vi "IIR Filter Design.vi"() -> ()   [LabVIEW 2020]
doc: "Displays the Transfer Function of the filter selected from the front panel controls. \n\nYou can select any of the 5 IIR filter design methods (Bessel, Butterworth, Chebyshev I and II, and Elliptic) and the passband type (lowpass, highpass, bandpass, and bandstop)."
uses:
  <vilib>/Analysis/3filter.llb/Filter Passband Type.ctl
  <vilib>/Utility/error.llb/DialogType.ctl
  <vilib>/Analysis/NI_AALPro.lvlib
  <vilib>/measure/NI_MAPro.lvlib
  <vilib>/Analysis/NI_AALBase.lvlib
panel:
  out "Error Message":string
  in  "filter type":T1
  in  "Stop":bool
  in  "sampling rate":dbl=1000.0 format="%#.6g"
  in  "Attenuation":dbl(slide)=40.0 scale=0.0..150.0
  in  "Ripple":dbl(slide)=0.1 scale=0.0..1.0
  in  "high cutoff frequency":dbl(slide)=300.0 scale=0.0..500.0
  in  "low cutoff frequency":dbl(slide)=100.0 scale=0.0..500.0
  in  "Order":i32(slide)=4 scale=0.0..10.0
  in  "Filter Design":T2(ring)
  out "Phase Response":cluster{dbl, dbl, dbl[]}(graph)
  out "Magnitude Response":cluster{dbl, dbl, dbl[]}(graph)
  # "Overview: Demonstrates the design options for IIR filters.\nRequirements: LabVIEW Full Development System\nInstructions:\n1. Run the VI.\n2. Manipulate the parameters and observe the results in the Magnitude Response and Phase Response graphs.\n3. Click Stop to stop the VI."
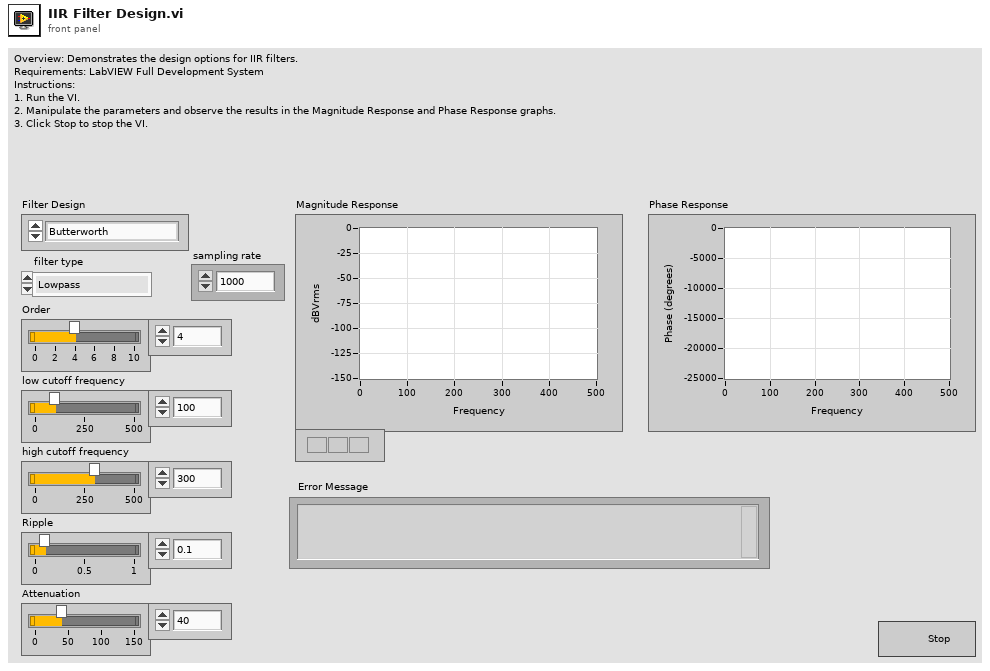
[diagram p1: front panel]
types:
  T1 = typedef "NI_AALBase.lvlib/Filter Passband Type.ctl" = enum32{"Lowpass", "Highpass", "Bandpass", "Bandstop"}
  T2 = enum16{"Butterworth", "Chebyshev", "Inverse Chebyshev", "Elliptic", "Bessel"}
  T3 = enum32{"Vrms", "Vpk", "Vrms^2", "Vpk^2", "Vrms/rtHz", "Vpk/rtHz", "Vrms^2/Hz", "Vpk^2/Hz"}
  T4 = enum16{"Power (Vrms^2)", "Amplitude (Vrms)", "Gain (amplitude ratio)"}
  T5 = typedef "DialogType.ctl" = u16
  T6 = cluster{"filter structure":enum32{"IIR 2nd Order", "IIR 4th Order"}, "Reverse Coefficients":dbl[], "Forward Coefficients":dbl[]}
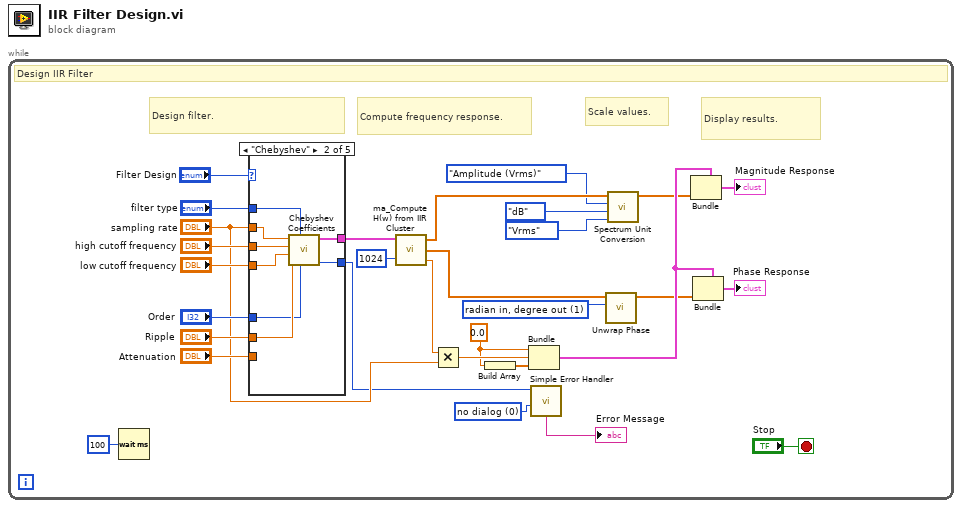
[diagram p0: block diagram]
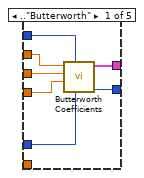
[diagram p2: hidden frame]
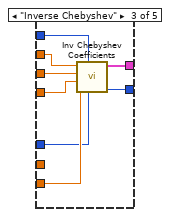
[diagram p3: hidden frame]
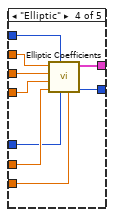
[diagram p4: hidden frame]
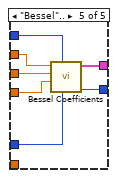
[diagram p5: hidden frame]
diagram:
  n1 = while {
    stop <- "Stop" stop-if-true
    w1 = 0.0
    w3 = T5 0 items=["no dialog", "OK message", "continue or stop message", "OK message + warnings", "continue/stop + warnings"] ("type of dialog (OK msg:1)")
    w10 = 1 items=["radian in, radian out", "radian in, degree out", "degree in, degree out", "degree in, radian out"] ("phase unit")
    # "Display results."
    # "Scale values."
    # "Compute frequency response."
    # "Design filter."
    # "Design IIR Filter"
    n2 = Wait (ms)(milliseconds to wait=u32 100) -> ()  [unwired: 1 out]
    n3 = case shown="\"Chebyshev\"" "Filter Design" {
      tunnel: "filter type" -> [w32 w45 w53 w60 w69]
      tunnel: "high cutoff frequency" -> [w37 w44 w52 w62 w68]
      tunnel: "low cutoff frequency" -> [w36 w43 w51 w61 w67]
      tunnel: "Order" -> [w35 w41 w49 w57 w66]
      tunnel: "Ripple" -> [_ w42 _ w59 _]
      tunnel: "Attenuation" -> [_ _ w50 w56 _]
      tunnel: "sampling rate" -> [w34 w40 w48 w58 w65]
      tunnel: [w33 w39 w47 w55 w64] -> w14
      tunnel: [w31 w38 w46 w54 w63] -> w2
      frame .."Butterworth" {
        n4 = call <vilib>:"Butterworth Coefficients.vi"("order"=w35, "filter type"=w32, "low cutoff freq: fl"=w36, "high cutoff freq: fh"=w37, "sampling freq: fs"=w34) -> ("error"=w31:i32, "IIR Filter Cluster"=w33:T6)  [unwired: 5 in]
      }
      frame "Chebyshev" {
        n5 = call <vilib>:"Chebyshev Coefficients.vi"("order"=w41, "filter type"=w45, "ripple(dB)"=w42, "low cutoff freq: fl"=w43, "high cutoff freq: fh"=w44, "sampling freq: fs"=w40) -> ("error"=w38:i32, "IIR Filter Cluster"=w39:T6)  [unwired: 4 in]
      }
      frame "Inverse Chebyshev" {
        n6 = call <vilib>:"Inv Chebyshev Coefficients.vi"("order"=w49, "filter type"=w53, "attenuation (dB)"=w50, "low cutoff freq: fl"=w51, "high cutoff freq: fh"=w52, "sampling freq: fs"=w48) -> ("error"=w46:i32, "IIR Filter Cluster"=w47:T6)  [unwired: 4 in]
      }
      frame "Elliptic" {
        n7 = call <vilib>:"Elliptic Coefficients.vi"("stopband attenuation (dB)"=w56, "order"=w57, "filter type"=w60, "passband ripple (dB)"=w59, "low cutoff freq: fl"=w61, "high cutoff freq: fh"=w62, "sampling freq: fs"=w58) -> ("error"=w54:i32, "IIR Filter Cluster"=w55:T6)  [unwired: 3 in]
      }
      frame "Bessel".. {
        n8 = call <vilib>:"Bessel Coefficients.vi"("order"=w66, "filter type"=w69, "low cutoff freq: fl"=w67, "high cutoff freq: fh"=w68, "sampling freq: fs"=w65) -> ("error"=w63:i32, "IIR Filter Cluster"=w64:T6)  [unwired: 5 in]
      }
    }
    n9 = call <vilib>:"ma_Compute H(w) from IIR Cluster.vi"("IIR Filter Cluster"=w14, "FFT size"=1024) -> ("Mag H(w)"=w13:dbl[], "Phase H(w)"=w11:dbl[], "df"=w5:dbl)
    n10 = Multiply(x=w5, y="sampling rate") -> (x*y=w26:dbl)
    n11 = Build Array ("array")(w1) -> (w25:dbl[])
    n12 = Bundle(w1, w26, w25) -> (w30:cluster{dbl, dbl, dbl[]})  [unwired: 1 in]
    n13 = call <vilib>:"Simple Error Handler.vi"("error code (no error:0)"=w2, "type of dialog (OK msg:1)"=w3) -> ("message"=→"Error Message":string)  [unwired: 3 in, 4 out]
    n14 = call <vilib>:"Unwrap Phase.vi"("phase unit"=w10, "Phase"=w11) -> ("Unwrapped Phase"=w29:dbl[])  [unwired: 8 in, 1 out]
    n15 = call <vilib>:"Spectrum Unit Conversion.vi"("display unit"=T3."Vrms", "log/linear"=enum16{"Linear", "dB", "dBm"}."dB", "spectrum type"=T4."Amplitude (Vrms)", "Spectrum in"=w13) -> ("Spectrum out"=w12:dbl[])  [unwired: 6 in, 1 out]
    n16 = Bundle(cluster=w30, w12) -> (→"Magnitude Response":cluster{dbl, dbl, dbl[]})  [unwired: 2 in]
    n17 = Bundle(cluster=w30, w29) -> (→"Phase Response":cluster{dbl, dbl, dbl[]})  [unwired: 2 in]
  }
